vi "Avantes - AVS_GetList.vi"(8 "error in (no error)":errorcluster, 10 "Sphere Indicator":T1, 11 "AVS Settings In":T2) -> (0 "error out":errorcluster, 3 "AVS Settings Out":T2)   [LabVIEW 2014, in "AvaSpec.lvlib" / "Avantes Spectrometer Functions.lvlib"]
uses:
  Avantes Spectrometer Functions.lvlib
  AVS settings.ctl
  Acquisition/Sphere Indicator.ctl
  AvaSpec.lvlib
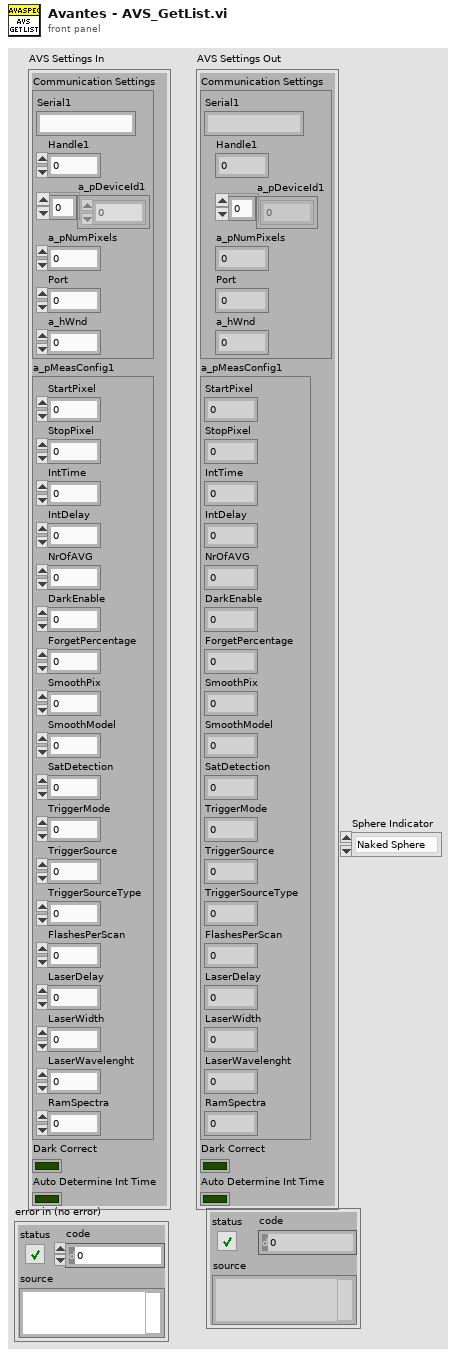
[diagram p1: front panel]
types:
  T1 = typedef "AvaSpec.lvlib/Sphere Indicator.ctl" = enum16{"Naked Sphere", "Insulated Sphere"}
  T2 = typedef "AvaSpec.lvlib/AVS settings.ctl" = cluster{"Communication Settings":cluster{"Serial1":string, "Handle1":i32, "a_pDeviceId1":u8[], "a_pNumPixels":u16, "Port":i32, "a_hWnd":i32}, "a_pMeasConfig1":cluster{"StartPixel":u16, "StopPixel":u16, "IntTime":sgl, "IntDelay":u32, "NrOfAVG":u32, "DarkEnable":u8, "ForgetPercentage":u8, "SmoothPix":u16, "SmoothModel":u8, "SatDetection":u8, "TriggerMode":u8, "TriggerSource":u8, "TriggerSourceType":u8, "FlashesPerScan":u16, "LaserDelay":u32, "LaserWidth":u32, "LaserWavelenght":sgl, "RamSpectra":u16}, "Dark Correct":bool, "Auto Determine Int Time":bool}
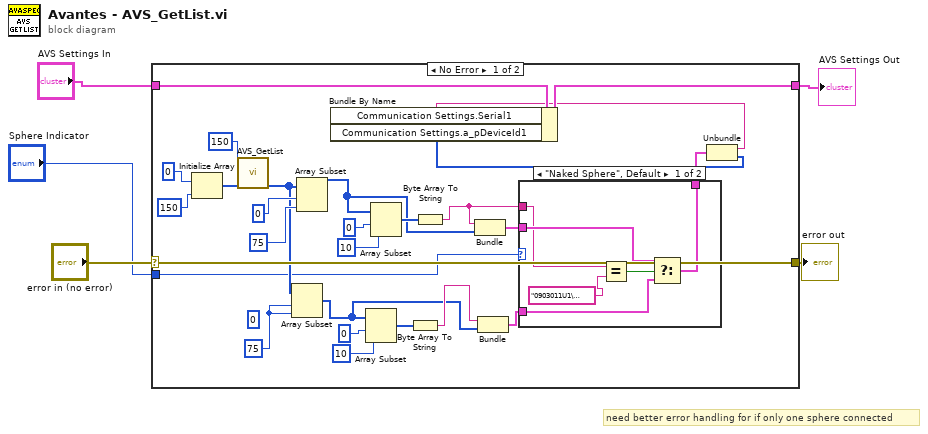
[diagram p0: block diagram]
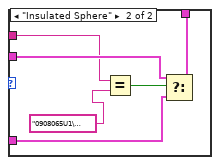
[diagram p2: hidden frame]
diagram:
  # "need better error handling for if only one sphere connected"
  n1 = case shown="No Error" "error in (no error)" {
    selector: "error in (no error)" -> [w32 w46]
    tunnel: [w21 w45] -> w2
    tunnel: "AVS Settings In" -> [w22 w45]
    tunnel: [w32 w46] -> w4
    tunnel: "Sphere Indicator" -> [w15 _]
    frame No Error {
      w17 = 75 ("length")
      (unwired) 0 ("index")
      n2 = Initialize Array(i8 0 ("element"), 150 ("dimension size")) -> (w28:i8[])
      n3 = call "AVS_GetList.vi"("ListSizeInput"=u32 150, "ListInpit"=w28) -> ("List Output"=w16:u8[])  [unwired: 11 in, 2 out]
      n4 = Array Subset(array=w16, index=w17, length=w17) -> (w13:u8[])
      n5 = Array Subset(array=w16, index=0, length=75) -> (w11:u8[])
      n6 = Array Subset(array=w13, index=0, length=10) -> (w20:u8[])
      n7 = Array Subset(array=w11, index=0, length=10) -> (w23:u8[])
      n8 = Byte Array To String(unsigned byte array=w20) -> (string=w14:string)
      n9 = Byte Array To String(unsigned byte array=w23) -> (string=w6:string)
      n10 = Bundle("string"=w6, w11) -> (w10:cluster{"string":string, u8[]})  [unwired: 1 in]
      n11 = Bundle("string"=w14, w13) -> (w12:cluster{"string":string, u8[]})  [unwired: 1 in]
      n12 = case shown="\"Naked Sphere\", Default" w15 {
        tunnel: w12 -> [w36 w42]
        tunnel: w10 -> [w37 w41]
        tunnel: [w35 w43] -> w9
        tunnel: w6 -> [w34 w40]
        frame "Naked Sphere", Default {
          n13 = Equal?(x=w34, y="0903011U1\u0000" ("string")) -> (x = y?=w38:bool)
          n14 = Select(t=w37, s=w38, f=w36) -> (s? t:f=w35:cluster{"string":string, u8[]})
        }
        frame "Insulated Sphere" {
          n15 = Equal?(x=w40, y="0908065U1\u0000" ("string")) -> (x = y?=w44:bool)
          n16 = Select(t=w41, s=w44, f=w42) -> (s? t:f=w43:cluster{"string":string, u8[]})
        }
      }
      n17 = Unbundle(w9) -> ("string"=w8:string, w7:u8[])
      n18 = Bundle By Name(cluster=w22, "Communication Settings.Serial1"=w8, "Communication Settings.a_pDeviceId1"=w7) -> (w21:T2)
    }
    frame Error {
    }
  }
  "error out" <- w4
  "AVS Settings Out" <- w2
